vi "Helm Heading PID Cycle.vi"(8 "error in (no error)":errorcluster, 11 "RDS Helm Actor in":refnum<class "RDS Helm Actor.lvclass">) -> (0 "error out":errorcluster, 3 "RDS Helm Actor out":refnum<class "RDS Helm Actor.lvclass">)   [LabVIEW 2015, in "RDS Helm Actor.lvlib" / "RDS Helm Actor.lvclass"]
uses:
  RDS Helm Actor.lvclass
  RDS Helm Actor.lvclass/RDS Helm Actor.ctl
  <vilib>/addons/control/pid/pid.llb/PID (DBL).vi
  <vilib>/addons/control/pid/NI_PID_pid.lvlib
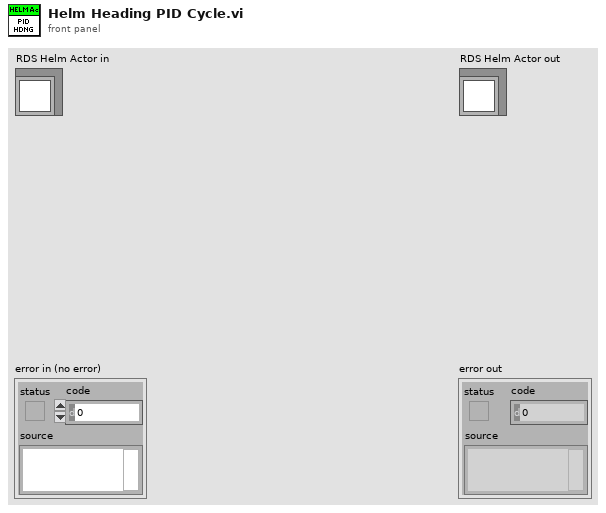
[diagram p1: front panel]
types:
  T1 = typedef "RDS Child Messages.lvlib/PID Gains Control.ctl" = cluster{"P (Kc)":sgl, "I (Ti)":sgl, "D (Td)":sgl}
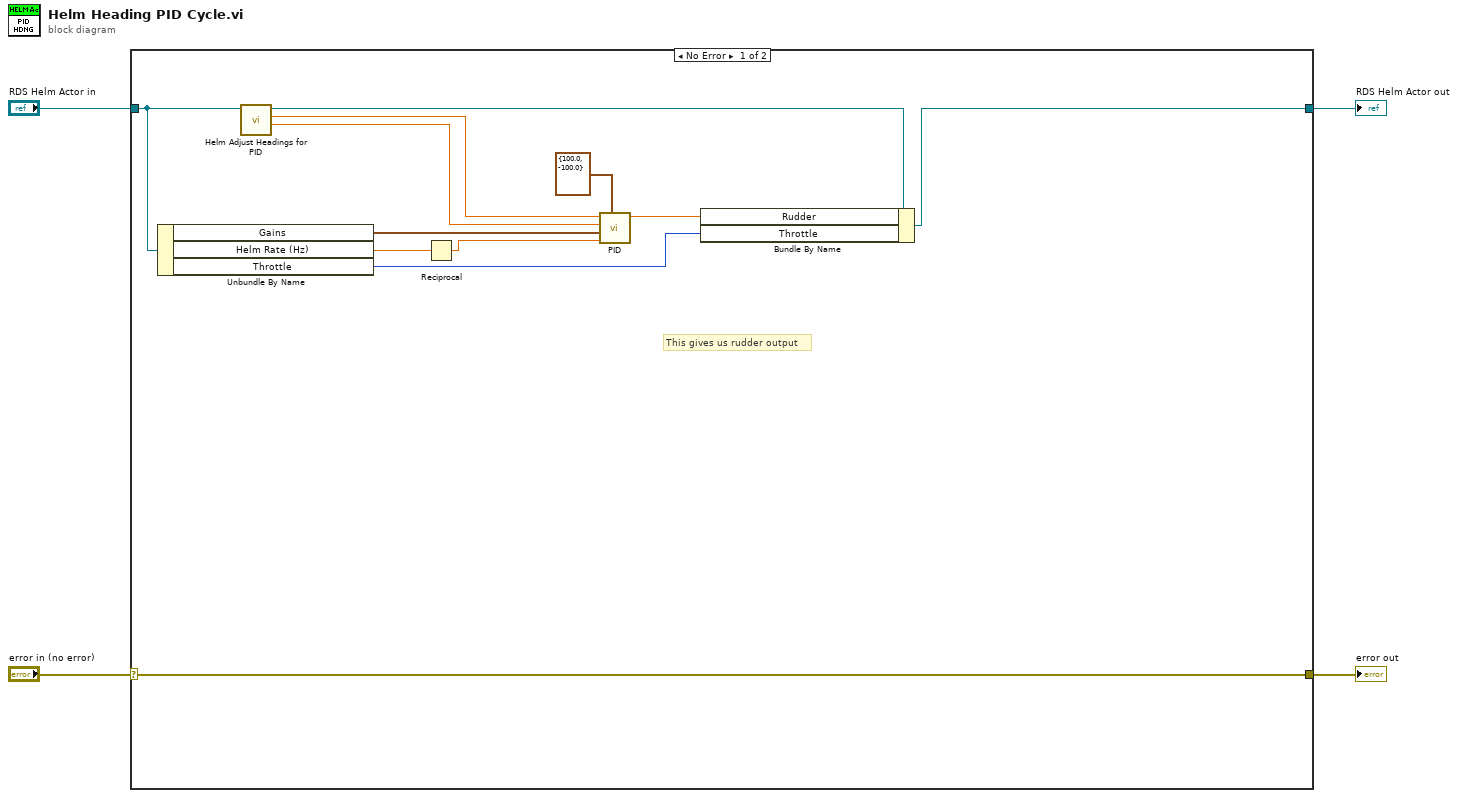
[diagram p0: block diagram]
diagram:
  n1 = case shown="No Error" "error in (no error)" {
    selector: "error in (no error)" -> [w16 w18]
    tunnel: [w16 w18] -> w3
    tunnel: [w5 w17] -> w1
    tunnel: "RDS Helm Actor in" -> [w12 w17]
    frame No Error {
      # "This gives us rudder output"
      n2 = Unbundle By Name(w12) -> ("Gains"=w11:T1, "Helm Rate (Hz)"=w10:sgl, "Throttle"=w7:i16)
      n3 = call "Helm Adjust Headings for PID.vi"("RDS Helm Actor in"=w12) -> ("Current Position"=w14:dbl, "Setpoint"=w15:dbl, "RDS Helm Actor out"=w6:refnum<class "RDS Helm Actor.lvclass">)  [unwired: 7 in, 1 out]
      n4 = Reciprocal(x=w10) -> (1/x=w9:sgl)
      n5 = call-poly <vilib>:"PID.vi"("output range"=cluster{"output high":dbl, "output low":dbl} {"output high"=100.0, "output low"=-100.0}, "dt (s)"=w9, "PID gains"=w11, "process variable"=w14, "setpoint"=w15) -> ("output"=w8:dbl)  [unwired: 5 in, 1 out]
      n6 = Bundle By Name(cluster=w6, "Rudder"=w8, "Throttle"=w7) -> (w5:refnum<class "RDS Helm Actor.lvclass">)
    }
    frame Error {
    }
  }
  "error out" <- w3
  "RDS Helm Actor out" <- w1
